vi "KeyB2901A_from Kei24xx.vi"() -> ()   [LabVIEW 2014]
uses:
  <vilib>/Utility/file.llb/Write To Spreadsheet File (string).vi
panel:
  in  "stop":bool
  in  "Source Mode  (0: Voltage)":u16(ring) items=["Voltage", "Current"]
  in  "VISA resource name 2":refnum<visa-resource-name>
  in  "Файл записи замеров":path
  in  "Ограничение":dbl format="%.2f"
  out "Замер":string
  in  "Выход":dbl
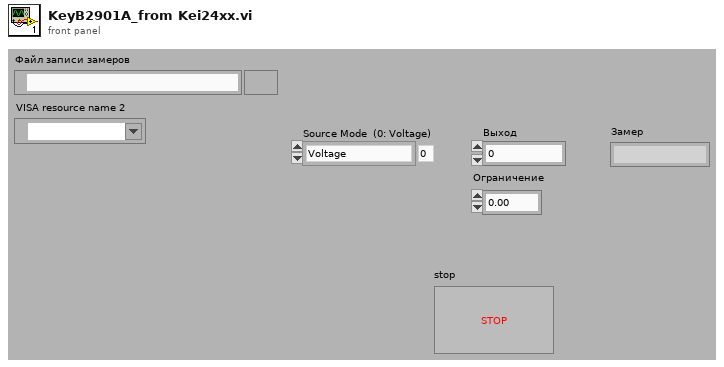
[diagram p1: front panel]
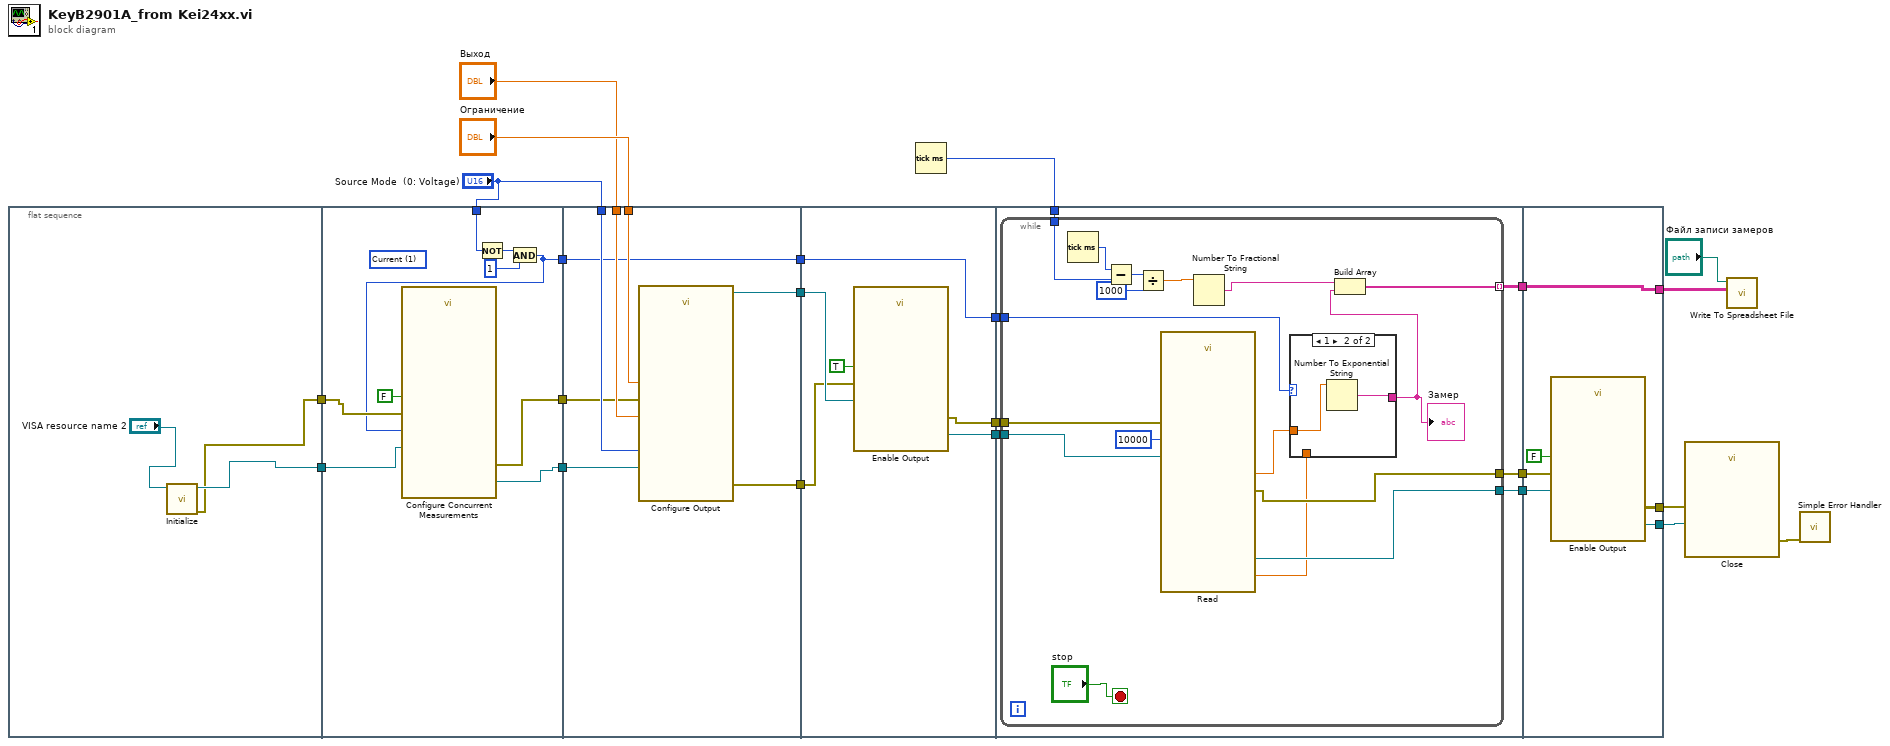
[diagram p0: block diagram]
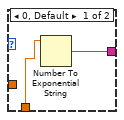
[diagram p2: hidden frame]
diagram:
  n1 = flat-sequence {
    tunnel: [w25] -> w8
    tunnel: [w24] -> w6
    tunnel: w8 -> [w33]
    tunnel: [w34] -> w7
    tunnel: w6 -> [w32]
    tunnel: [w35] -> w5
    tunnel: "Source Mode  (0: Voltage)" -> [w30]
    tunnel: [w27] -> w1
    tunnel: "Ограничение" -> [w43]
    tunnel: "Выход" -> [w42]
    tunnel: "Source Mode  (0: Voltage)" -> [w41]
    tunnel: w7 -> [w40]
    tunnel: w5 -> [w39]
    tunnel: [w38] -> w21
    tunnel: [w37] -> w20
    tunnel: [w36] -> w3
    tunnel: w1 -> [w36]
    tunnel: w21 -> [w49]
    tunnel: w20 -> [w48]
    tunnel: [w46] -> w19
    tunnel: [w45] -> w18
    tunnel: w3 -> [w44]
    tunnel: [w44] -> w2
    tunnel: w19 -> [w56]
    tunnel: w18 -> [w55]
    tunnel: w17 -> [w54]
    tunnel: [w53] -> w14
    tunnel: [w52] -> w13
    tunnel: [w51] -> w12
    tunnel: w2 -> [w50]
    tunnel: [w83] -> w15
    tunnel: w14 -> [w83]
    tunnel: w13 -> [w81]
    tunnel: w12 -> [w80]
    tunnel: [w79] -> w11
    tunnel: [w78] -> w10
    frame #0 {
      n2 = call "Initialize.vi"("VISA resource name"="VISA resource name 2") -> ("error out"=w24:errorcluster, "VISA resource name out"=w25:refnum<visa-resource-name>)  [unwired: 9 in]
    }
    frame #1 {
      (unwired) u16 1 items=["Volts", "Current", "Resistance", "Volt, Current", "Volts, Resistance", "Current, Resistance", "All"] ("Measurement Selection (3: Volts, Current)")
      n3 = Not(x=w30) -> (.not. x?=w29:u16)
      n4 = And(x=w29, y=u16 1) -> (x .and. y?=w27:u16)
      n5 = call "Configure Concurrent Measurements.vi"("error in (no error)"=w32, "Measurement Selection (3: Volts, Current)"=w27, "Enable Concurrent Measurements (F: Disable)"=FALSE, "VISA resource name"=w33) -> ("error out"=w35:errorcluster, "VISA resource name out"=w34:refnum<visa-resource-name>)  [unwired: 6 in]
    }
    frame #2 {
      n6 = call "Configure Output.vi"("Source Mode  (0: Voltage)"=w41, "error in (no error)"=w39, "Compliance  Level (0.1)"=w43, "Output Level (0)"=w42, "VISA resource name"=w40) -> ("error out"=w37:errorcluster, "VISA resource name out"=w38:refnum<visa-resource-name>)  [unwired: 5 in]
    }
    frame #3 {
      n7 = call "Enable Output.vi"("error in (no error)"=w48, "Enable Output (T: Enable)"=TRUE, "VISA resource name"=w49) -> ("error out"=w46:errorcluster, "VISA resource name out"=w45:refnum<visa-resource-name>)  [unwired: 7 in]
    }
    frame #4 {
      n8 = while {
        tunnel: w56 -> [w72]
        tunnel: w55 -> [w71]
        tunnel: w54 -> [w66]
        tunnel: [w61] -> w53 mode=indexing
        tunnel: [w64] -> w52
        tunnel: [w63] -> w51
        tunnel: w50 -> [w60]
        stop <- "stop" stop-if-true
        n9 = Tick Count (ms)() -> (millisecond timer value=w70:u32)
        n10 = Subtract(x=w70, y=w66) -> (x-y=w69:u32)
        n11 = Divide(x=w69, y=u32 1000) -> (x/y=w67:dbl)
        n12 = call-poly "Read.vi"("VISA resource name"=w71, "Timeout (10000 ms)"=10000, "error in (no error)"=w72) -> ("Voltage"=w58:sgl, "VISA resource name out"=w64:refnum<visa-resource-name>, "Current"=w59:sgl, "error out"=w63:errorcluster)  [unwired: 6 in, 3 out]
        n13 = Number To Fractional String(number=w67) -> (F-format string=w65:string)  [unwired: 3 in]
        n14 = case shown="1" w60 {
          tunnel: w59 -> [_ w77]
          tunnel: w58 -> [w75 _]
          tunnel: [w74 w76] -> w57
          frame 0, Default {
            n15 = Number To Exponential String(number=w75) -> (E-format string=w74:string)  [unwired: 3 in]
          }
          frame 1 {
            n16 = Number To Exponential String(number=w77) -> (E-format string=w76:string)  [unwired: 3 in]
          }
        }
        "Замер" <- w57
        n17 = Build Array(w65, w57) -> (w61:string[])
      }
    }
    frame #5 {
      n18 = call "Enable Output.vi"("error in (no error)"=w80, "Enable Output (T: Enable)"=FALSE, "VISA resource name"=w81) -> ("error out"=w79:errorcluster, "VISA resource name out"=w78:refnum<visa-resource-name>)  [unwired: 7 in]
    }
  }
  n19 = Tick Count (ms)() -> (millisecond timer value=w17:u32)
  n20 = call "Close.vi"("error in (no error)"=w11, "VISA resource name"=w10) -> ("error out"=w9:errorcluster)  [unwired: 9 in]
  n21 = call-poly <vilib>:"Write To Spreadsheet File.vi"("2D data"=w15, "file path (dialog if empty)"="Файл записи замеров") -> ()  [unwired: 6 in, 1 out]
  n22 = call <vilib>:"Simple Error Handler.vi"("error in (no error)"=w9) -> ()  [unwired: 4 in, 5 out]
